vi "Write Setting.vi"(8 "error in (no error)":errorcluster, 10 "Setting":u8[](array[numeric]), 11 "Update U8 Array in":refnum<class "Update U8 Array.lvclass">) -> (0 "error out":errorcluster, 3 "Update U8 Array out":refnum<class "Update U8 Array.lvclass">)   [LabVIEW 2014, in "Update U8 Array.lvclass"]
uses:
  Update U8 Array.lvclass
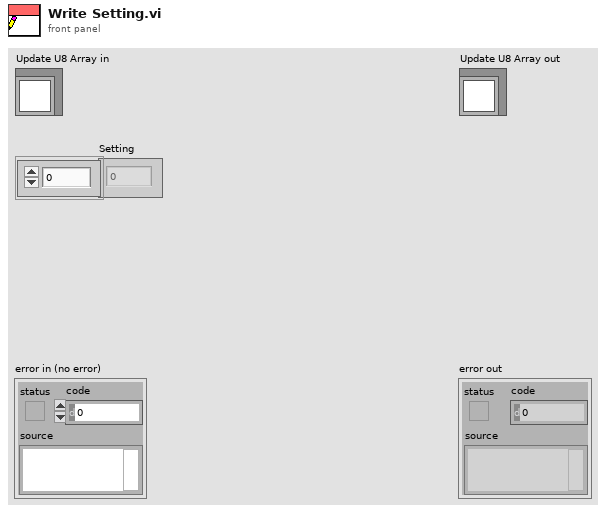
[diagram p1: front panel]
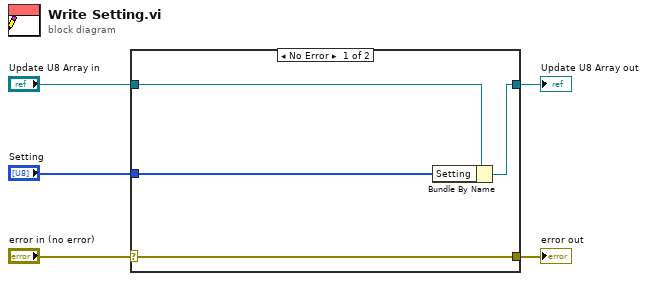
[diagram p0: block diagram]
diagram:
  n1 = case shown="No Error" "error in (no error)" {
    selector: "error in (no error)" -> [w9 w10]
    tunnel: [w9 w10] -> w4
    tunnel: [w7 w11] -> w2
    tunnel: "Update U8 Array in" -> [w8 w11]
    tunnel: "Setting" -> [w6 _]
    frame No Error {
      n2 = Bundle By Name(cluster=w8, "Setting"=w6) -> (w7:refnum<class "Update U8 Array.lvclass">)
    }
    frame Error {
    }
  }
  "error out" <- w4
  "Update U8 Array out" <- w2
